vi "Close Error Log.vi"(8 "Error In":errorcluster) -> (0 "Error Out":errorcluster)   [LabVIEW 2023, in "Error Manager.lvlib" / "Error Log.lvclass"]
uses:
  Error Log Ref (library variable).vi
  Error Log.lvclass
  Error Log.lvclass/Error Log.ctl
panel:
  # "Input\nInputs to the VI"
  # "Development\nControls or indicators that are useful for development or testing, but which are not outputs of the VI."
  # "Output\nOutputs of the VI"
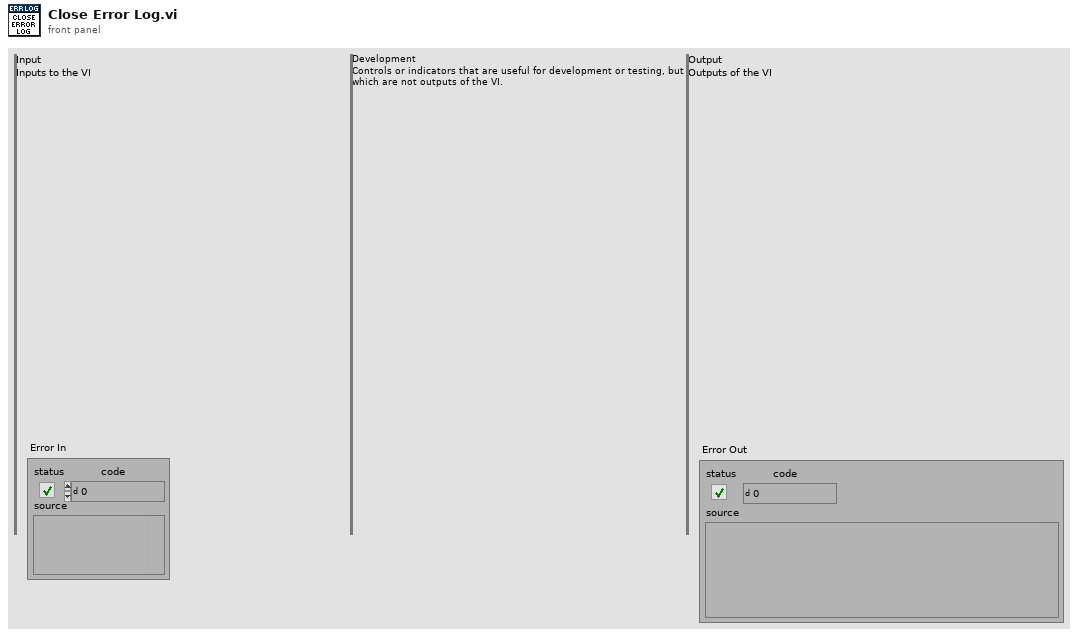
[diagram p1: front panel]
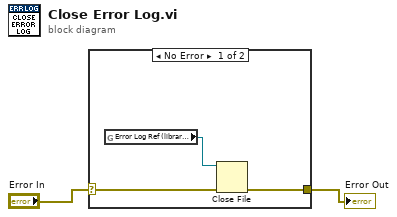
[diagram p0: block diagram]
diagram:
  n1 = case shown="No Error" "Error In" {
    selector: "Error In" -> [w5 w6]
    tunnel: [w4 w6] -> w1
    frame No Error {
      n2 = global read "Error Log Ref (library variable).vi" item#0() -> (w3:refnum<file>)
      n3 = Close File(refnum=w3, error in=w5) -> (error out=w4:errorcluster)  [unwired: 1 out]
    }
    frame Error {
    }
  }
  "Error Out" <- w1
